vi "(Sub_VI)_Control_tabs_AOs_ini.vi"(0 "Physical Channels":tag="DAQ_Rex/ao0", 2 "Package for PID":T1, 3 "Sti. Gal 2 AOs Ctr Term (PFI2)":tag, 5 "error in":errorcluster) -> (6 "task out":refnum<k21>, 8 "error out":errorcluster)   [LabVIEW 2012]
doc: "I. Description:\nThis example demonstrates how to continuously output a waveform using an internal sample clock. The automatic regeneration of data has been disabled, so new data has to be provided throughout the duration of the continuous Analog Output operation. This allows the generation of any arbitrary frequency as this VI computes new data for each iteration of the loop, maintaining phase continuity of the signal. The regeneration of data has also been adjusted so that the newest data is output as quickly as possible; thus reducing the lag between the changing of the data and the output of that data.\n\nII. Instructions for Running:\n1. Select the Physical Channel to correspond to where your signal is output on the DAQ device.\n2. Enter the Minimum and Maximum Voltage range.\n3. Specify the desired Sample Clock Rate of the output Waveform. Higher sample clock rates will produce a smoother waveform.\n4. Manually specify the Analog Output buffer size, in number of samples. A larger buffer would help non-regenerative operations avoid errors due to occasional high CPU load. \nNote: \nThe Analog Output buffer has to be at least as big as the amount of data being written to the board per iteration. The recommended buffer size would be at least twice the amount of data being written to the board per iteration.\n5. Enter the Waveform Information. See the documentation of the Basic Function Generator SubVI for information on each parameter.\n\nIII. Block Diagram Steps:\n1. Create an Analog Output Voltage channel.\n2. Configure the task to prohibit the automatic regeneration of data.\n2a. Set the transfer condition to Less than Full. Allows for more rapid updates of Output Buffer.\n3. Call the DAQmx (Sample Clock) VI to set the sample clock rate. Additionally, set the sample mode to Continuous.\n4. Read the actual sample clock rate (eventually coerced depending on the hardware used). \n5. Compute the desired waveform, using the buffer size and the actual update rate. This VI keeps track of the phase of the waveform to ensure that the generated signal is continuous.\n6. Write the waveform to the output buffer. \n7a. Call the Start VI. This is only needed when the loop is executed for the first time.\n7b. Do nothing.\n8. Loop continuously until user presses the Stop button. Every iteration computes and writes a new waveform to the buffer.\n9. Call the Clear Task VI to clear the Task.\n10. Use the popup dialog box to display an error or warning if any.\n\nIV. I/O Connections Overview:\nMake sure your signal output terminal matches the Physical Channel I/O Control. For further connection information, refer to your hardware reference manual."
uses:
  <vilib>/DAQmx/write.llb/DAQmx Write (Analog 2D DBL NChan NSamp).vi
  <vilib>/DAQmx/create/channels.llb/DAQmx Create Channel (AO-Voltage-Basic).vi
  <vilib>/DAQmx/configure/timing.llb/DAQmx Timing (Sample Clock).vi
  <vilib>/DAQmx/miscellaneous.llb/DAQmx Fill In Error Info.vi
  <resource>/objmgr/daqmx.rc
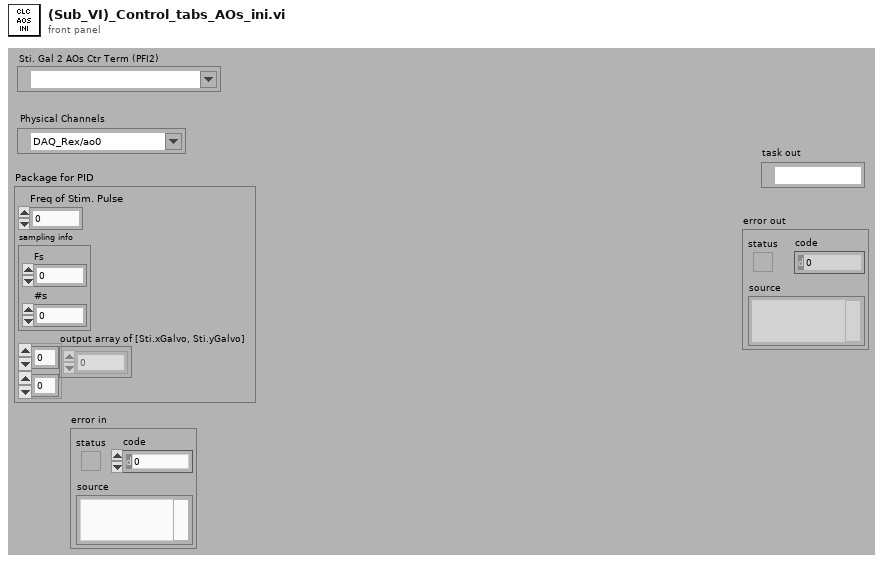
[diagram p1: front panel]
types:
  T1 = cluster{"Freq of Stim. Pulse":dbl, "sampling info":cluster{"Fs":dbl, "#s":dbl}, "output array of [Sti.xGalvo, Sti.yGalvo]":dbl[][]}
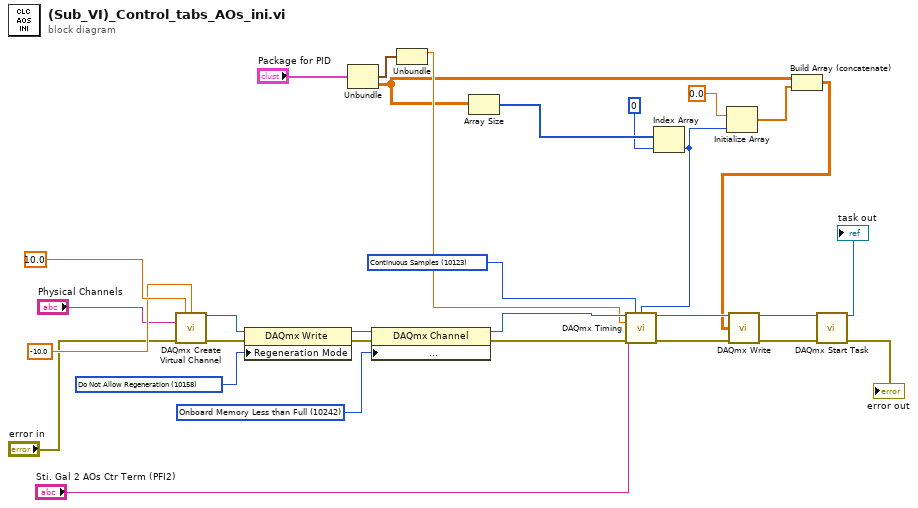
[diagram p0: block diagram]
diagram:
  w19 = 10242 items=["Onboard Memory Empty"=10235, "Onboard Memory Half Full or Less"=10239, "Onboard Memory Less than Full"=10242] ("AO.DataXferReqCond")
  w26 = 10158 items=["Allow Regeneration"=10097, "Do Not Allow Regeneration"=10158] ("RegenMode")
  w30 = 10123 items=["Finite Samples"=10178, "Continuous Samples"=10123] ("sample mode")
  n1 = call-poly <vilib>:"DAQmx Create Virtual Channel.vi"("maximum value"=10.0 ("Maximum Value"), "minimum value"=-10.0 ("Minimum Value"), "physical channels"="Physical Channels", "error in"="error in") -> ("task out"=w25:refnum<k21>, "error out"=w24:errorcluster)  [unwired: 10 in]
  n2 = property class="DAQmx Write"(reference=w25, error in=w24, "Regeneration Mode"=w26) -> (reference out=w23:refnum<k21>, error out=w20:errorcluster)
  n3 = Unbundle("Package for PID") -> ("sampling info"=w7:cluster{"Fs":dbl, "#s":dbl}, "output array of [Sti.xGalvo, Sti.yGalvo]"=w3:dbl[][])  [unwired: 1 out]
  n4 = property class="DAQmx Channel"(reference=w23, error in=w20, "Analog Output:General Properties:Advanced:Data Transfer and Memory:Data Transfer Request Condition"=w19) -> (reference out=w22:refnum<k21>, error out=w21:errorcluster)
  n5 = Unbundle(w7) -> ("Fs"=w6:dbl)  [unwired: 1 out]
  n6 = Array Size(array=w3) -> (size(s)=w13:i32[])
  n7 = Index Array(array=w13, index=0) -> (element=w4:i32)
  n8 = call-poly <vilib>:"DAQmx Timing.vi"("task/channels in"=w22, "sample mode"=w30, "samples per channel"=w4, "rate"=w6, "source"="Sti. Gal 2 AOs Ctr Term (PFI2)", "error in"=w21) -> ("task out"=w15:refnum<k21>, "error out"=w14:errorcluster)  [unwired: 8 in]
  n9 = Initialize Array(0.0 ("element"), w4) -> (w2:dbl[])
  n10 = Build Array (concatenate)(w3, w2) -> (w1:dbl[][])
  n11 = call-poly <vilib>:"DAQmx Write.vi"("task/channels in"=w15, "data"=w1, "error in"=w14) -> ("task out"=w16:refnum<k21>, "error out"=w17:errorcluster)  [unwired: 10 in, 1 out]
  n12 = call <vilib>:"DAQmx Start Task.vi"("task/channels in"=w16, "error in"=w17) -> ("task out"=→"task out":refnum<k21>, "error out"=→"error out":errorcluster)  [unwired: 12 in]
